vi "Robot Main.vi"() -> ()   [LabVIEW 2016]
doc: "This VI implements the framework and scheduler for your robotics program. It should not be necessary to modify the framework. You are expected to add your code to the VIs called from Robot Main - the ones located in the Team Code folder within the project."
uses:
  Vision Server/typedef/Vision Control Type.ctl
  Vision Server/Vision Server.lvclass
panel:
  in  "set?":bool
  in  "stop":bool
  in  "Vision Mode":T1
  in  "error in":errorcluster
  out "error out":errorcluster
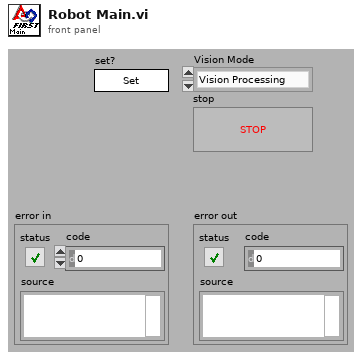
[diagram p1: front panel]
types:
  T1 = typedef "Vision Server.lvclass/Vision Control Type.ctl" = enum16{"Vision Processing", "Driver Assistance"}
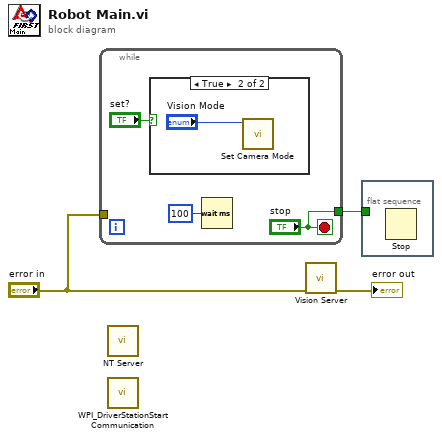
[diagram p0: block diagram]
diagram:
  n1 = while {
    tunnel: "error in" -> [_]
    tunnel: ["stop"] -> w1
    stop <- "stop" stop-if-true
    n2 = case shown="True" "set?" {
      frame False {
      }
      frame True {
        n3 = call "Set Camera Mode.vi"("Vision Mode"="Vision Mode") -> ()  [unwired: 10 in, 1 out]
      }
    }
    n4 = Wait (ms)(milliseconds to wait=u32 100) -> ()  [unwired: 1 out]
  }
  n5 = call <vilib>:"NT Server.vi"() -> ()  [unwired: 12 in]
  n6 = call <vilib>:"WPI_DriverStationStart Communication.vi"() -> ()  [unwired: 2 in, 10 out]
  n7 = call "Vision Server.vi"("error in"="error in") -> ("error out"=→"error out":errorcluster)  [unwired: 10 in]
  n8 = flat-sequence {
    tunnel: w1 -> [_]
    frame #0 {
      n9 = Stop() -> ()  [unwired: 1 in]
    }
  }
